vi "Save Results.vi"(8 "error in (no error)":errorcluster, 10 "Results":refnum<class "Result.lvclass">[](array[class]), 11 "TestMonitor in":refnum<class "TestMonitor.lvclass">) -> (0 "error out":errorcluster, 3 "TestMonitor out":refnum<class "TestMonitor.lvclass">)   [LabVIEW 2018, in "TestMonitor.lvclass"]
doc: "This VI will take the array of results, format them and write them to the permanent report."
uses:
  TestMonitor.lvclass
  Result/Result.lvclass
  TestMonitor.lvclass/TestMonitor.ctl
  <vilib>/Skyline/TestMonitor/Test Step/Test Step Data.ctl
  <vilib>/Skyline/Utilities/Property.ctl
  <vilib>/Skyline/TestMonitor/Test Step/Create Test Step (Multiple).vi
  <vilib>/Skyline/TestMonitor/Test Step/NI SystemLink Test Step.lvclass
  <vilib>/Skyline/TestMonitor/Test Result/NI SystemLink Test Result.lvclass
  <vilib>/Skyline/Utilities/NI Skyline Utilities.lvlib
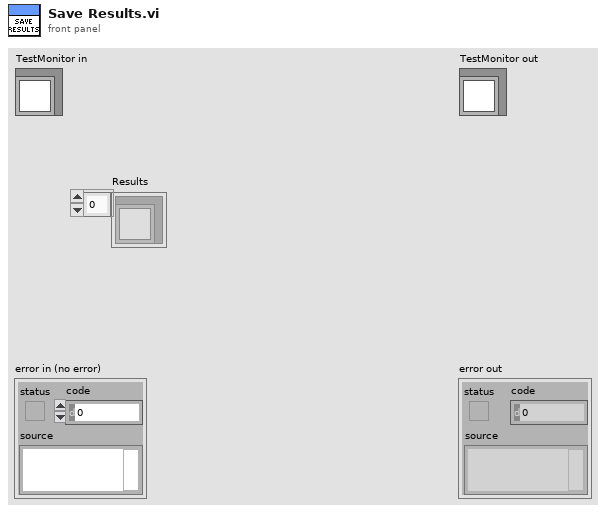
[diagram p1: front panel]
types:
  T1 = typedef "NI Skyline Utilities.lvlib/Property.ctl" = cluster{"key":string, "value":string}
  T2 = typedef "NI SystemLink Test Step.lvclass/Test Step Data.ctl" = cluster{"text":string, "parameters":cluster{"parameter list":T1[]}[]}
  T3 = typedef "Step.lvclass/Step Status.ctl" = enum16{"Start", "Passed", "Failed", "Error", "Done", "Terminated", "Skipped", "Running"}
  T4 = typedef "NI SystemLink Test Monitor.lvlib/Status Type.ctl" = enum16{"Failed", "Passed", "Looping", "Skipped", "Custom", "Done", "Running", "Waiting", "Terminated", "Errored", "Timed Out", "None"}
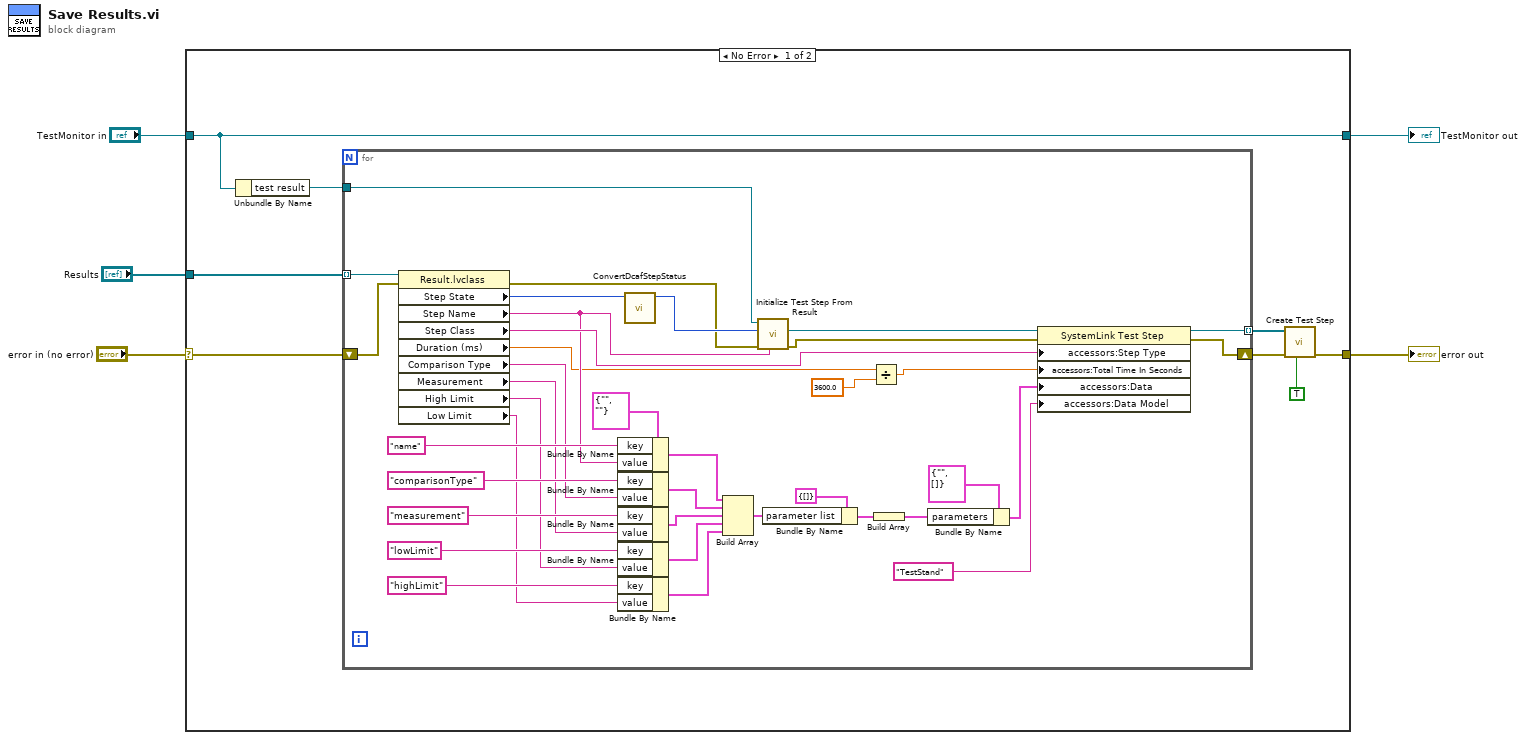
[diagram p0: block diagram]
diagram:
  n1 = case shown="No Error" "error in (no error)" {
    selector: "error in (no error)" -> [w13 w52]
    tunnel: [w9 w52] -> w5
    tunnel: [w7 w51] -> w3
    tunnel: "TestMonitor in" -> [w7 w51]
    tunnel: "Results" -> [w12 _]
    frame No Error {
      n2 = Unbundle By Name(w7) -> ("test result"=w6:refnum<class "NI SystemLink Test Result.lvclass">)
      n3 = for {
        shift-right: [w44] -> w10
        shift-left: w13 -> [w49]
        tunnel: w12 -> [w50] mode=indexing
        tunnel: [w45] -> w11 mode=indexing
        tunnel: w6 -> [w43]
        w15 = T1 {"key"="", "value"=""} ("property")
        n4 = property class="Result.lvclass"(reference=w50, error in=w49) -> (error out=w17:errorcluster, "Step State"=w46:T3, "Step Name"=w35:string, "Step Class"=w42:string, "Duration (ms)"=w20:dbl, "Comparison Type"=w21:string, "Measurement"=w31:string, "High Limit"=w30:string, "Low Limit"=w29:string)  [unwired: 1 out]
        n5 = Bundle By Name(cluster=w15, "key"="name", "value"=w35) -> (w28:T1)
        n6 = Bundle By Name(cluster=w15, "key"="comparisonType", "value"=w21) -> (w27:T1)
        n7 = Bundle By Name(cluster=w15, "key"="measurement", "value"=w31) -> (w26:T1)
        n8 = Bundle By Name(cluster=w15, "key"="lowLimit", "value"=w30) -> (w25:T1)
        n9 = Bundle By Name(cluster=w15, "key"="highLimit", "value"=w29) -> (w24:T1)
        n10 = call "ConvertDcafStepStatus.vi"("DCAF Step State"=w46) -> ("Systemlink Status"=w47:T4)  [unwired: 10 in]
        n11 = Build Array(w28, w27, w26, w25, w24) -> (w23:T1[])
        n12 = call <vilib>:"Initialize Test Step From Result.vi"("step name"=w35, "error in (no error)"=w17, "status type"=w47, "test result in"=w43) -> ("error out"=w16:errorcluster, "test step"=w48:refnum<class "NI SystemLink Test Step.lvclass">)  [unwired: 5 in, 1 out]
        n13 = Bundle By Name(cluster=cluster{"parameter list":T1[]} {"parameter list"=[]} ("element"), "parameter list"=w23) -> (w38:cluster{"parameter list":T1[]})
        n14 = Divide(x=w20, y=3600.0) -> (x/y=w19:dbl)
        n15 = Build Array(w38) -> (w39:cluster{"parameter list":T1[]}[])
        n16 = Bundle By Name(cluster=T2 {"text"="", "parameters"=[]} ("Data"), "parameters"=w39) -> (w22:T2)
        n17 = property class="SystemLink Test Step"(reference=w48, error in=w16, "accessors:Step Type"=w42, "accessors:Total Time In Seconds"=w19, "accessors:Data"=w22, "accessors:Data Model"="TestStand" ("Data Model")) -> (reference out=w45:refnum<class "NI SystemLink Test Step.lvclass">, error out=w44:errorcluster)
      }
      n18 = call-poly <vilib>:"Create Test Step.vi"("update result total time (F)"=TRUE, "error in (no error)"=w10, "test steps in"=w11) -> ("error out"=w9:errorcluster)  [unwired: 6 in, 2 out]
    }
    frame Error {
    }
  }
  "error out" <- w5
  "TestMonitor out" <- w3
